vi "LeftShiftRegister.vi"(8 "error in":errorcluster, 11 "reference":refnum<vi>) -> (0 "error out":errorcluster, 3 "ShiftRegister out":refnum<class "LeftShiftRegister.lvclass">)   [LabVIEW 2014, in "Raspberry Pi Compatible Compiler for LabVIEW.lvlib" / "LeftShiftRegister.lvclass"]
uses:
  LeftShiftRegister.lvclass
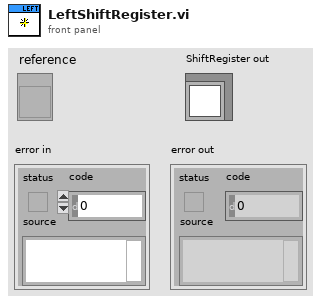
[diagram p1: front panel]
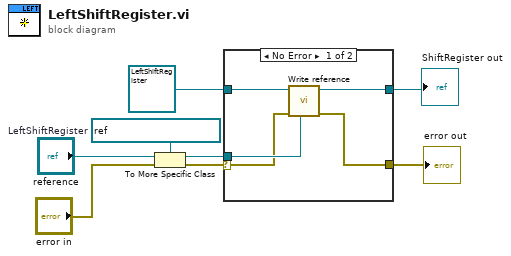
[diagram p0: block diagram]
diagram:
  w8 = refnum<vi> refnum  # LeftShiftRegister
  n1 = To More Specific Class(target class=w8, reference="reference", error in="error in") -> (specific class reference=w6:refnum<vi>, error out=w7:errorcluster)
  n2 = case shown="No Error" w7 {
    selector: w7 -> [w10 w14]
    tunnel: refnum<class "LeftShiftRegister.lvclass"> refnum ("ShiftRegister in") -> [w13 w15]
    tunnel: [w12 w15] -> w2
    tunnel: [w9 w14] -> w1
    tunnel: w6 -> [w11 _]
    frame No Error {
      n3 = call-dynamic "Write reference.vi"("reference"=w11, "error in"=w10, "GObject in"=w13) -> ("error out"=w9:errorcluster, "GObject out"=w12:refnum<class "LeftShiftRegister.lvclass">)  [unwired: 5 in]
    }
    frame Error {
    }
  }
  "error out" <- w1
  "ShiftRegister out" <- w2
